vi "冰箱运行流程.vi"   [LabVIEW 2016, in "环境动力单元.lvlib"]
uses:
  <vilib>/ptbypt/NI_PtbyPt.lvlib
types:
  T1 = cluster{"功能开关":enum16{"关闭", "开启"}, "开启时间":u16, "关闭时间":u16}
  T2 = typedef "LVDateTimeRec.ctl" = cluster{"秒数的小数部分":dbl, "秒":i32, "分":i32, "时":i32, "日":i32, "月":i32, "年":i32, "天数（周）":i32, "天数（年）":i32, "DST":i32}
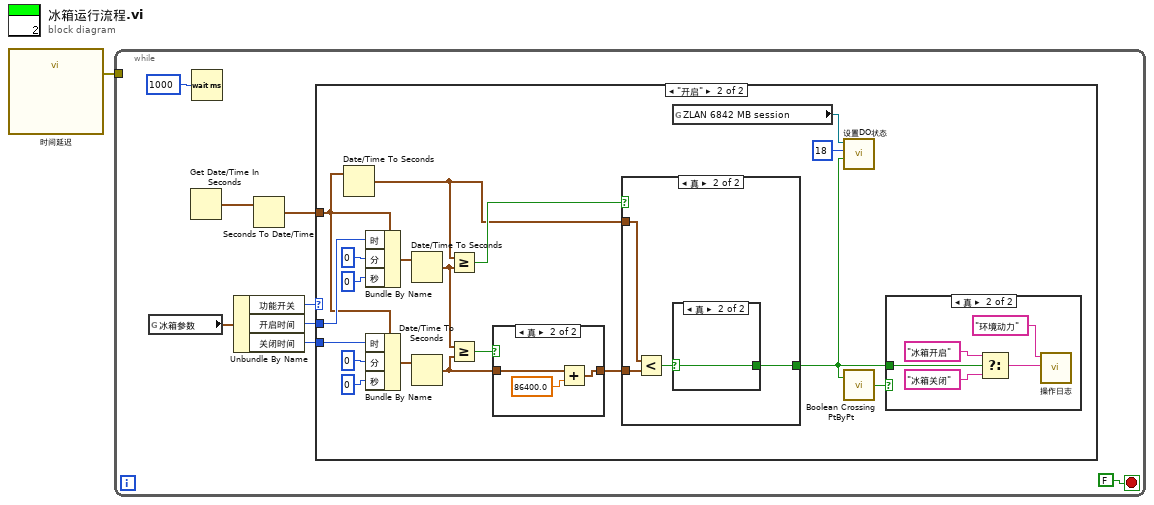
[diagram p0: block diagram]
diagram:
  n1 = call "时间延迟"() -> ("error out"=w1:errorcluster)  [unwired: 11 in]
  n2 = while {
    tunnel: w1 -> [_]
    stop <- FALSE stop-if-true
    n3 = global read "通讯全局变量断电保存.vi" "冰箱参数"() -> (w9:T1)
    n4 = Get Date/Time In Seconds() -> (seconds since 1Jan1904=w4:timestamp)
    n5 = Wait (ms)(milliseconds to wait=u32 1000 ("等待时间（毫秒）")) -> ()  [unwired: 1 out]
    n6 = Unbundle By Name(w9) -> ("功能开关"=w8:enum16{"关闭", "开启"}, "开启时间"=w7:u16, "关闭时间"=w6:u16)
    n7 = Seconds To Date/Time(time stamp (now)=w4) -> (date time rec=w5:T2)  [unwired: 1 in]
    n8 = case shown="\"开启\"" w8 {
      tunnel: w7 -> [_ w28]
      tunnel: w6 -> [_ w27]
      tunnel: w5 -> [_ w19]
      frame "关闭", Default {
      }
      frame "开启" {
        n9 = Date/Time To Seconds(2:w19) -> (0:w18:timestamp)  [unwired: 1 in]
        n10 = Bundle By Name(cluster=w19, "时"=w28, "分"=0, "秒"=0) -> (w22:T2)
        n11 = Bundle By Name(cluster=w19, "时"=w27, "分"=0, "秒"=0) -> (w21:T2)
        n12 = Date/Time To Seconds(2:w22) -> (0:w17:timestamp)  [unwired: 1 in]
        n13 = Date/Time To Seconds(2:w21) -> (0:w15:timestamp)  [unwired: 1 in]
        n14 = Greater Or Equal?(x=w18, y=w17) -> (x >= y?=w20:bool)
        n15 = Greater Or Equal?(x=w17, y=w15) -> (x >= y?=w16:bool)
        n16 = case shown="真" w16 {
          tunnel: w15 -> [w34 w37]
          tunnel: [w34 w36] -> w14
          frame False {
          }
          frame True {
            n17 = Add(x=w37, y=86400.0) -> (x+y=w36:timestamp)
          }
        }
        n18 = case shown="真" w20 {
          tunnel: w14 -> [_ w41]
          tunnel: w18 -> [_ w40]
          tunnel: [_ w38] -> w10
          frame False {
          }
          frame True {
            n19 = Less?(x=w40, y=w41) -> (x < y?=w39:bool)
            n20 = case shown="真" w39 {
              selector: w39 -> [_ w42]
              tunnel: [_ w42] -> w38
              frame False {
              }
              frame True {
              }
            }
          }
        }
        n21 = global read "通讯全局变量.vi" "ZLAN 6842 MB session"() -> (w12:refnum<class "MB_Master.lvclass">)
        n22 = call "设置DO状态.vi"("value"=w10, "address"=u16 18, "MB session in"=w12) -> ()  [unwired: 7 in, 2 out]
        n23 = call <vilib>:"Boolean Crossing PtByPt.vi"("input"=w10) -> ("crossing"=w11:bool)  [unwired: 2 in]
        n24 = case shown="真" w11 {
          tunnel: w10 -> [_ w32]
          frame False {
          }
          frame True {
            n25 = Select(t="冰箱开启" ("设备"), s=w32, f="冰箱关闭" ("设备")) -> (s? t:f=w29:string)
            n26 = call "操作日志.vi"("日志信息"=w29, "设备"="环境动力") -> ()  [unwired: 9 in, 1 out]
          }
        }
      }
    }
  }
